vi "GUI.vi"() -> ()   [LabVIEW 2024]
uses:
  vision/#AntennaControlNumber.ctl
  <vilib>/userDefined/High Color/IMAQdx.ctl
  <vilib>/sound2/lvsound2.llb/Sound Data Format.ctl
  dacAquisition/#AquisitionParameter.ctl
panel:
  in  "StartButton":bool
  in  "StopButton":bool
  in  "TabControl":enum32{"Setup", "Vision", "Correlation"}(tab)
  out "AudioGraph":dbl[](graph)
  in  "AquisitionParameters":T1={"SampleRate"=10000.0, "BufferSize"=512, "Channels"="cDAQ1Mod1/ai0:3"}
  in  "SoundFormat":T2={"sample rate (S/s)"=22050.0, "number of channels"=2, "bits per sample"=16}
  in  "Signal type":T3(ring)
  in  "Amplitude":dbl=1.0 format="%0.2f"
  in  "AudioBuffer":i32
  in  "MasterOffset":dbl(slide) scale=10.0..10000.0
  in  "ChannelBounds":T4(array[cluster])
  out "VideoAccuracy [mm/px]":dbl format="%_6g"
  out "Image":T5(plugin-control)
  out "FPS":dbl format="%.1f"
  in  "Reverse fingers":bool
  in  "SelectingButton":bool
  in  "Antenna":T6
  in  "TestVsion":bool caption="Blank Button"
  in  "Camera source":T7
  in  "AntDistance [mm]":dbl format="%_6g"
  out "VISION DISTANCES":sgl[][](graph)
  out "ANTENNAS DISTANCES":sgl[][](graph)
  out "XY Graph":cluster{dbl[], dbl[]}[](graph)
  out "Image 2":T5(plugin-control) caption="Image"
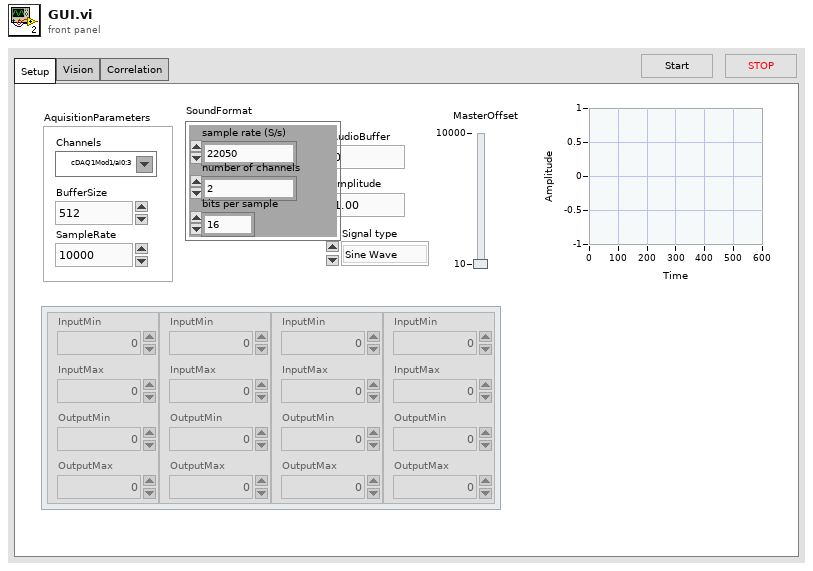
[diagram p1: front panel]
types:
  T1 = typedef "#AquisitionParameter.ctl" = cluster{"SampleRate":dbl, "BufferSize":i32, "Channels":tag}
  T2 = typedef "Sound Data Format.ctl" = cluster{"sample rate (S/s)":dbl, "number of channels":i32, "bits per sample":i32}
  T3 = enum16{"Sine Wave", "Triangle Wave", "Square Wave", "Sawtooth Wave"}
  T4 = cluster{"InputMin":dbl, "InputMax":dbl, "OutputMin":dbl, "OutputMax":dbl}[]
  T5 = typedef "IMAQ Image.ctl" = refnum<image>
  T6 = typedef "#AntennaControlNumber.ctl" = enum16{"Ant1", "Ant2", "Ant3", "Ant4"}
  T7 = typedef "IMAQdx.ctl" = refnum<k21>
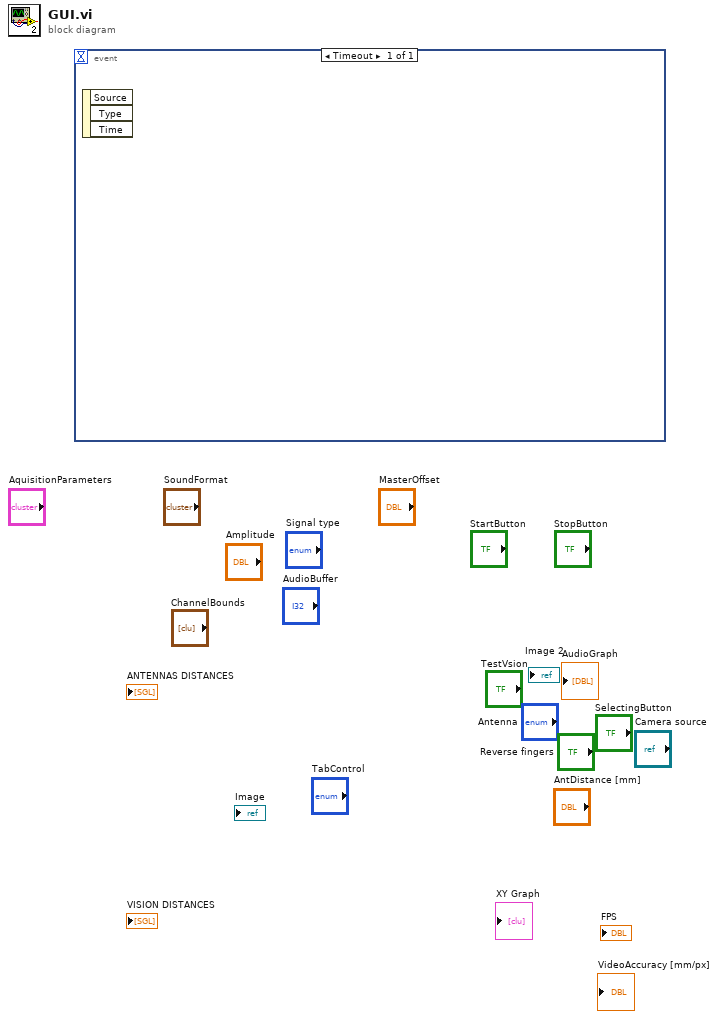
[diagram p0: block diagram]
diagram:
  n1 = event shown="[0] Timeout" {
    selector: _ -> [_]
    dyn-events: _ -> [_]
    timeout: _ -> [_]
    event Timeout {
      n2 = event-data() -> ()  [unwired: 1 in, 3 out]
    }
  }
